vi "ActiView806-Lores.vi"() -> ()   [LabVIEW 2020] (continued)
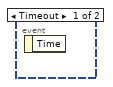
[diagram p2: hidden frame]
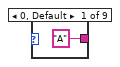
[diagram p3: hidden frame]
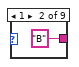
[diagram p4: hidden frame]
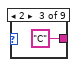
[diagram p5: hidden frame]
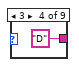
[diagram p6: hidden frame]
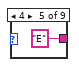
[diagram p7: hidden frame]
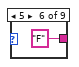
[diagram p8: hidden frame]
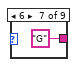
[diagram p9: hidden frame]
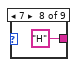
[diagram p10: hidden frame]
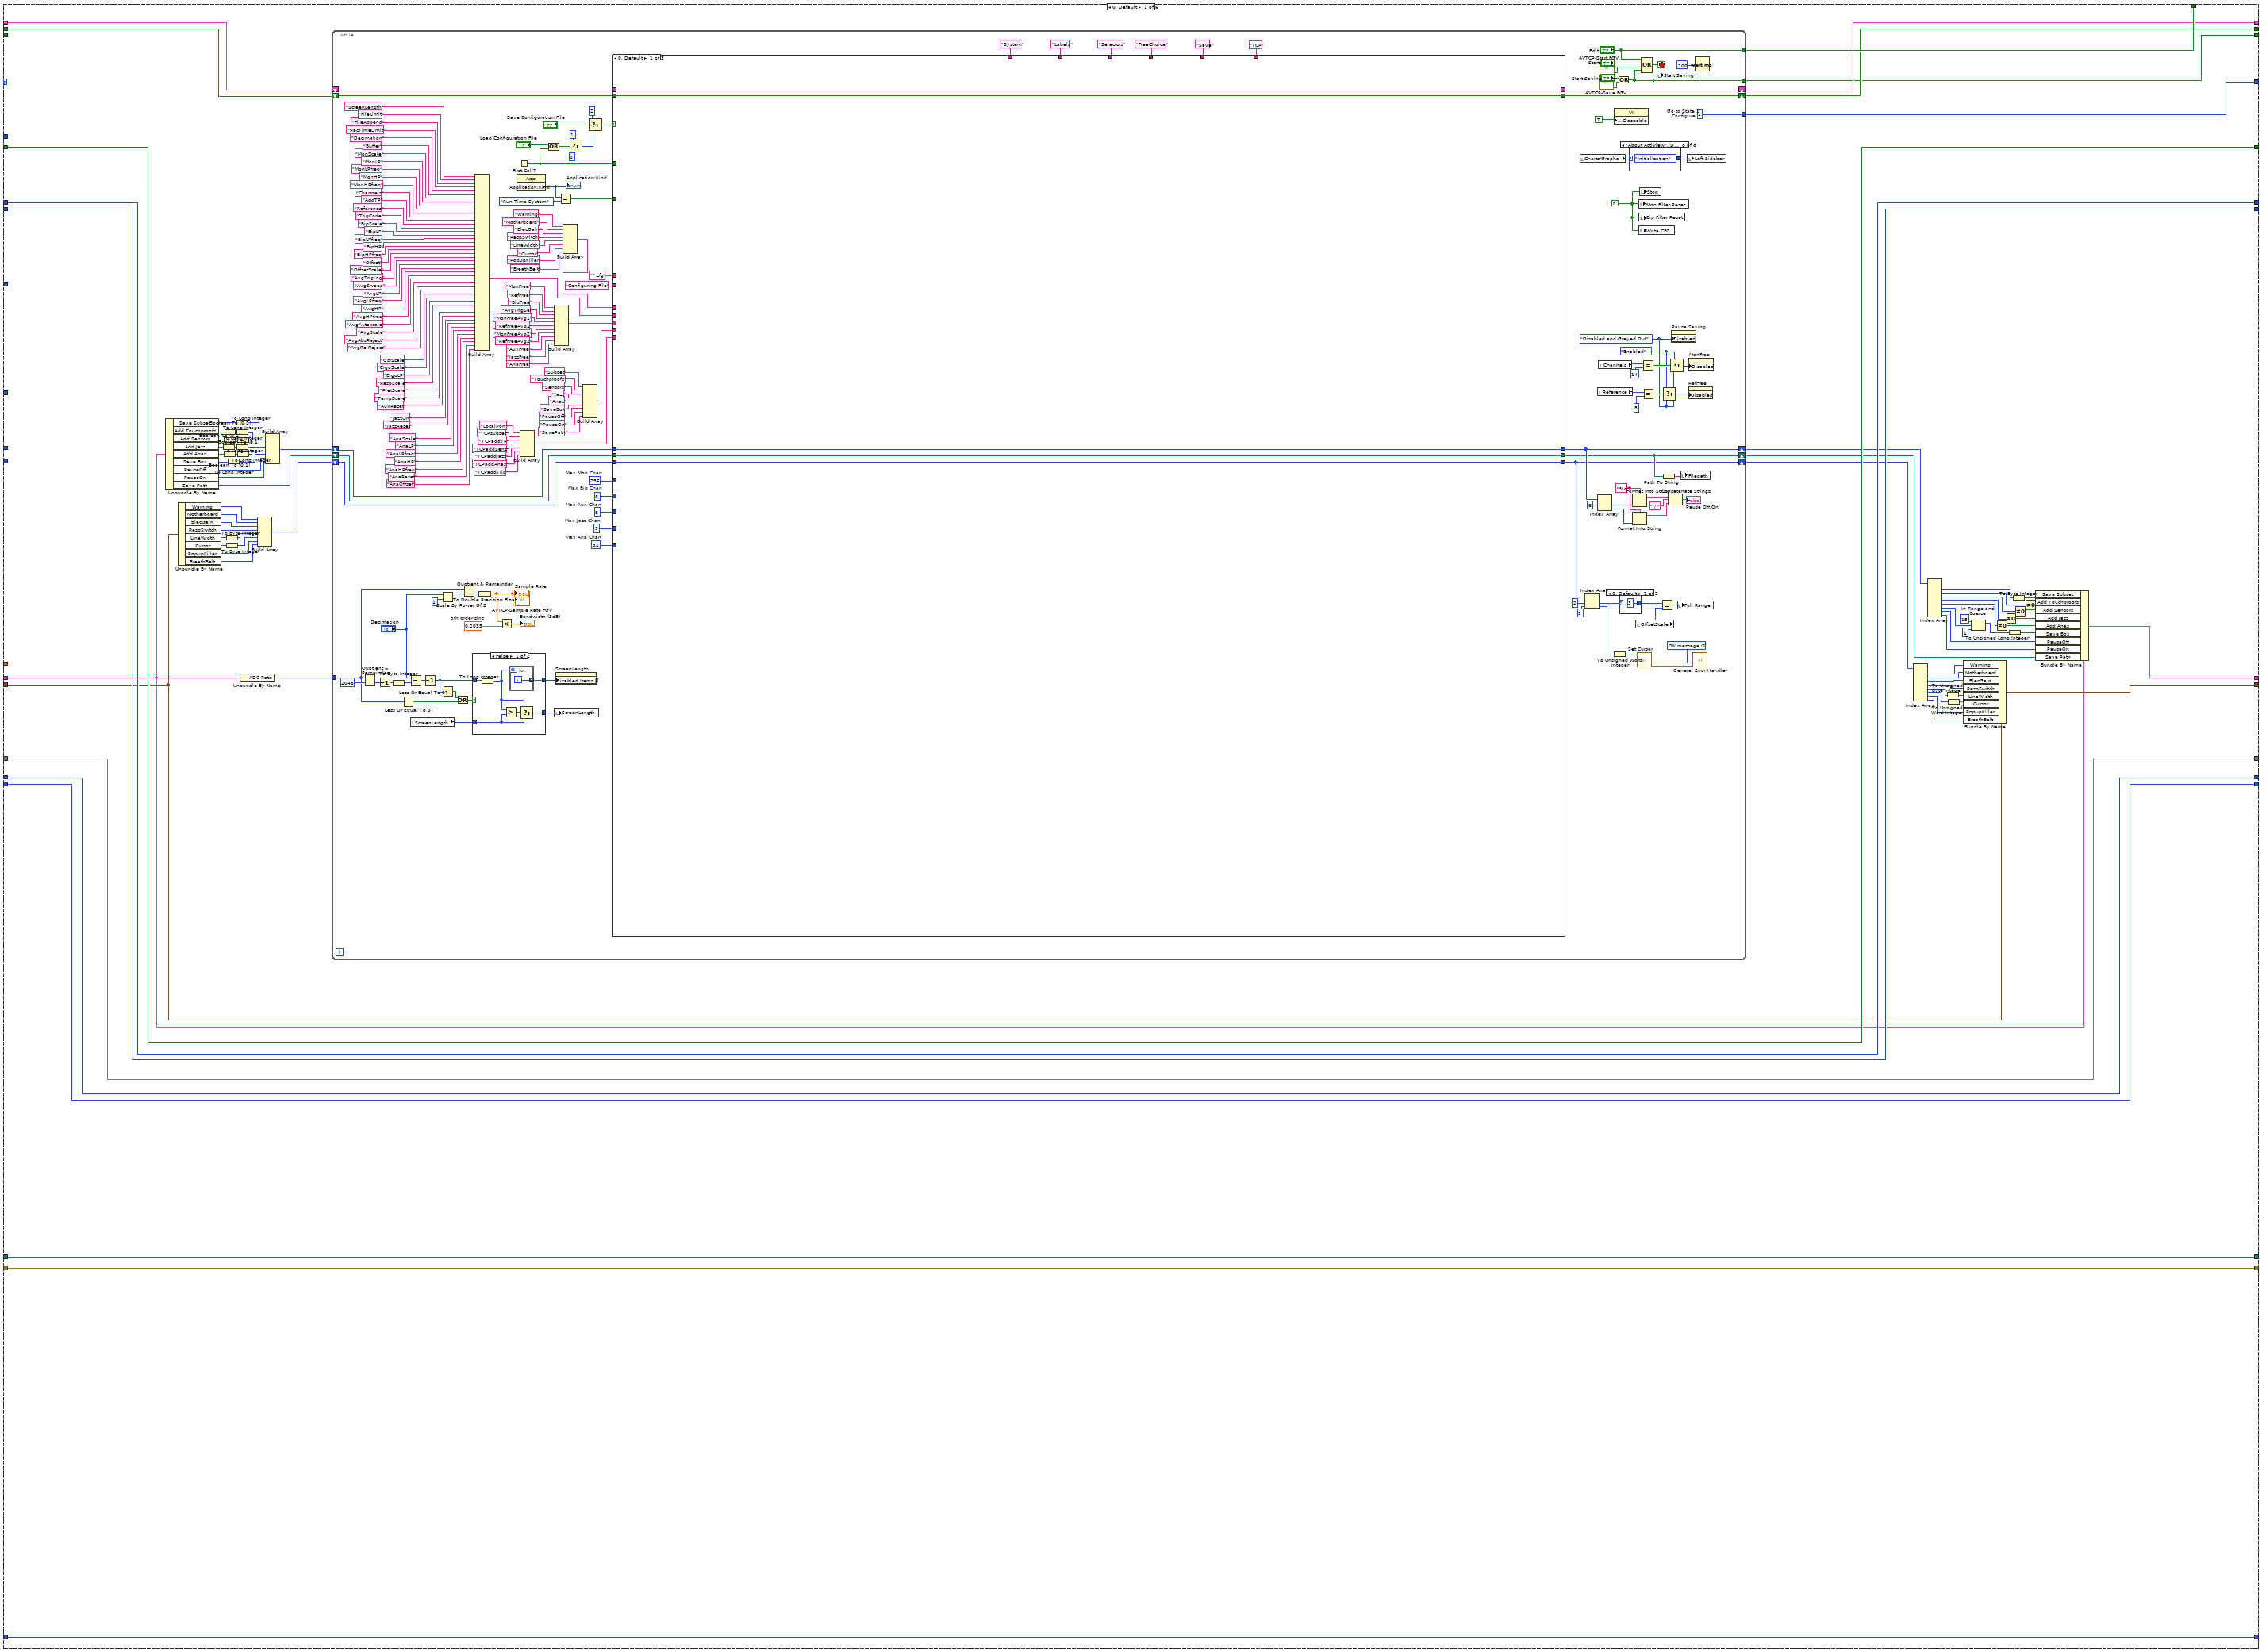
[diagram p11: hidden frame]
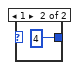
[diagram p12: hidden frame]
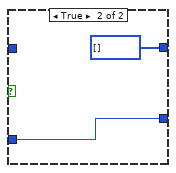
[diagram p13: hidden frame]
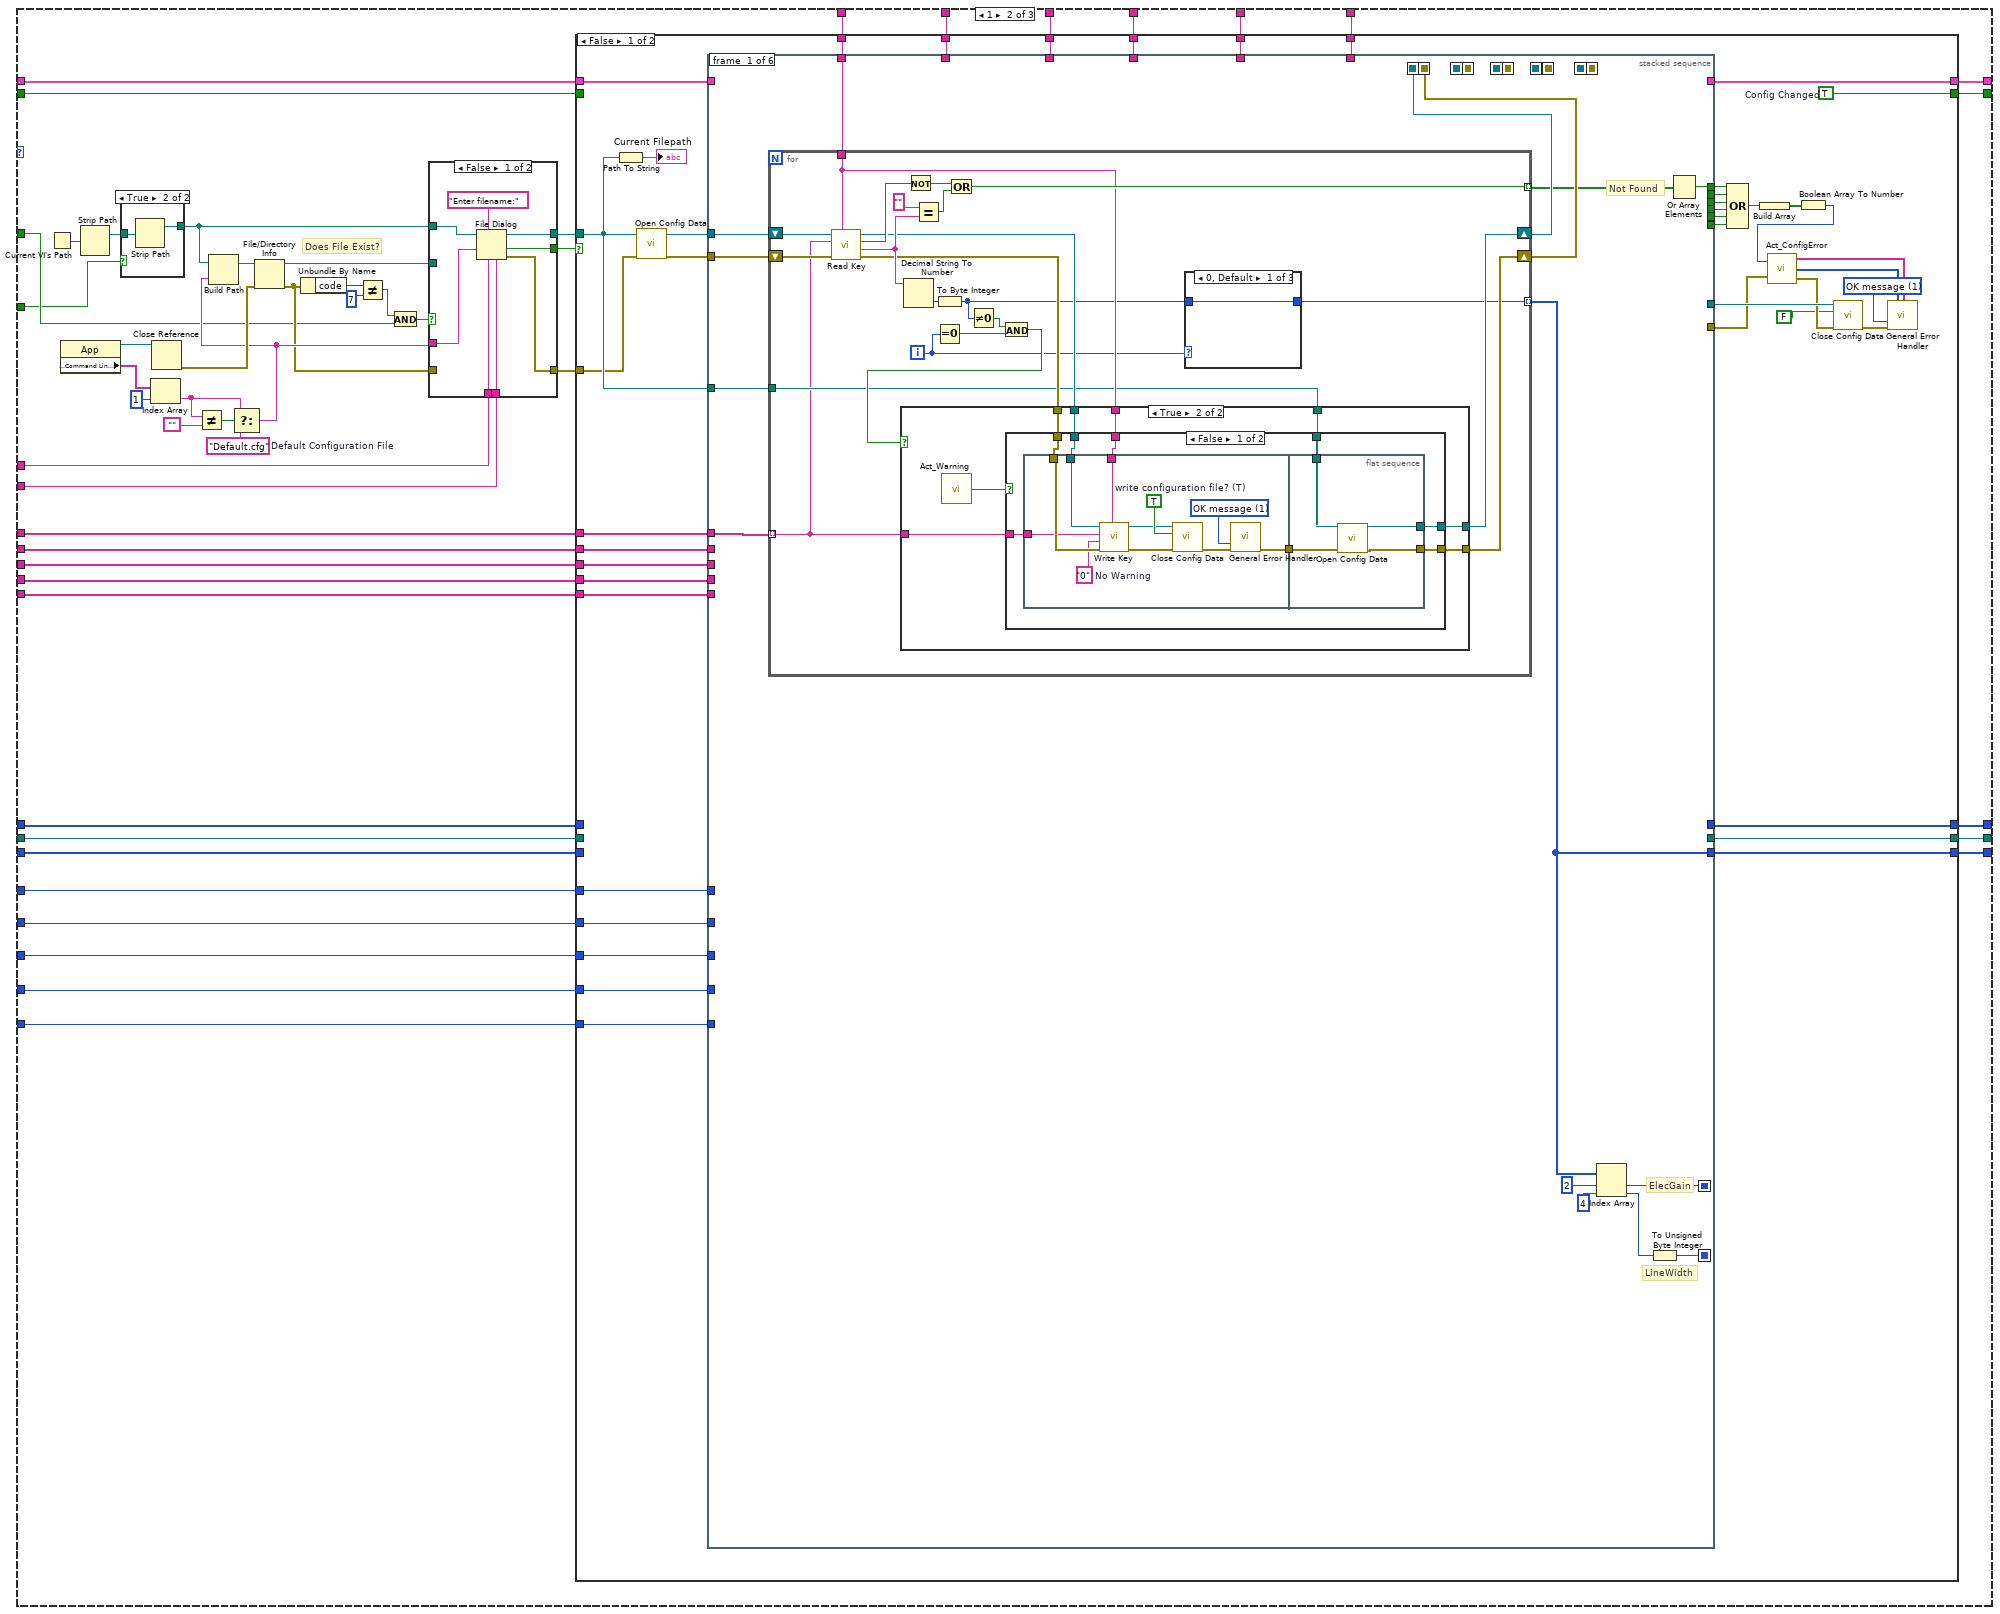
[diagram p14: hidden frame]
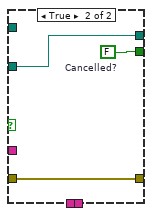
[diagram p15: hidden frame]
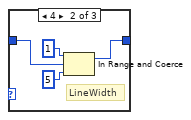
[diagram p16: hidden frame]
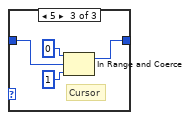
[diagram p17: hidden frame]
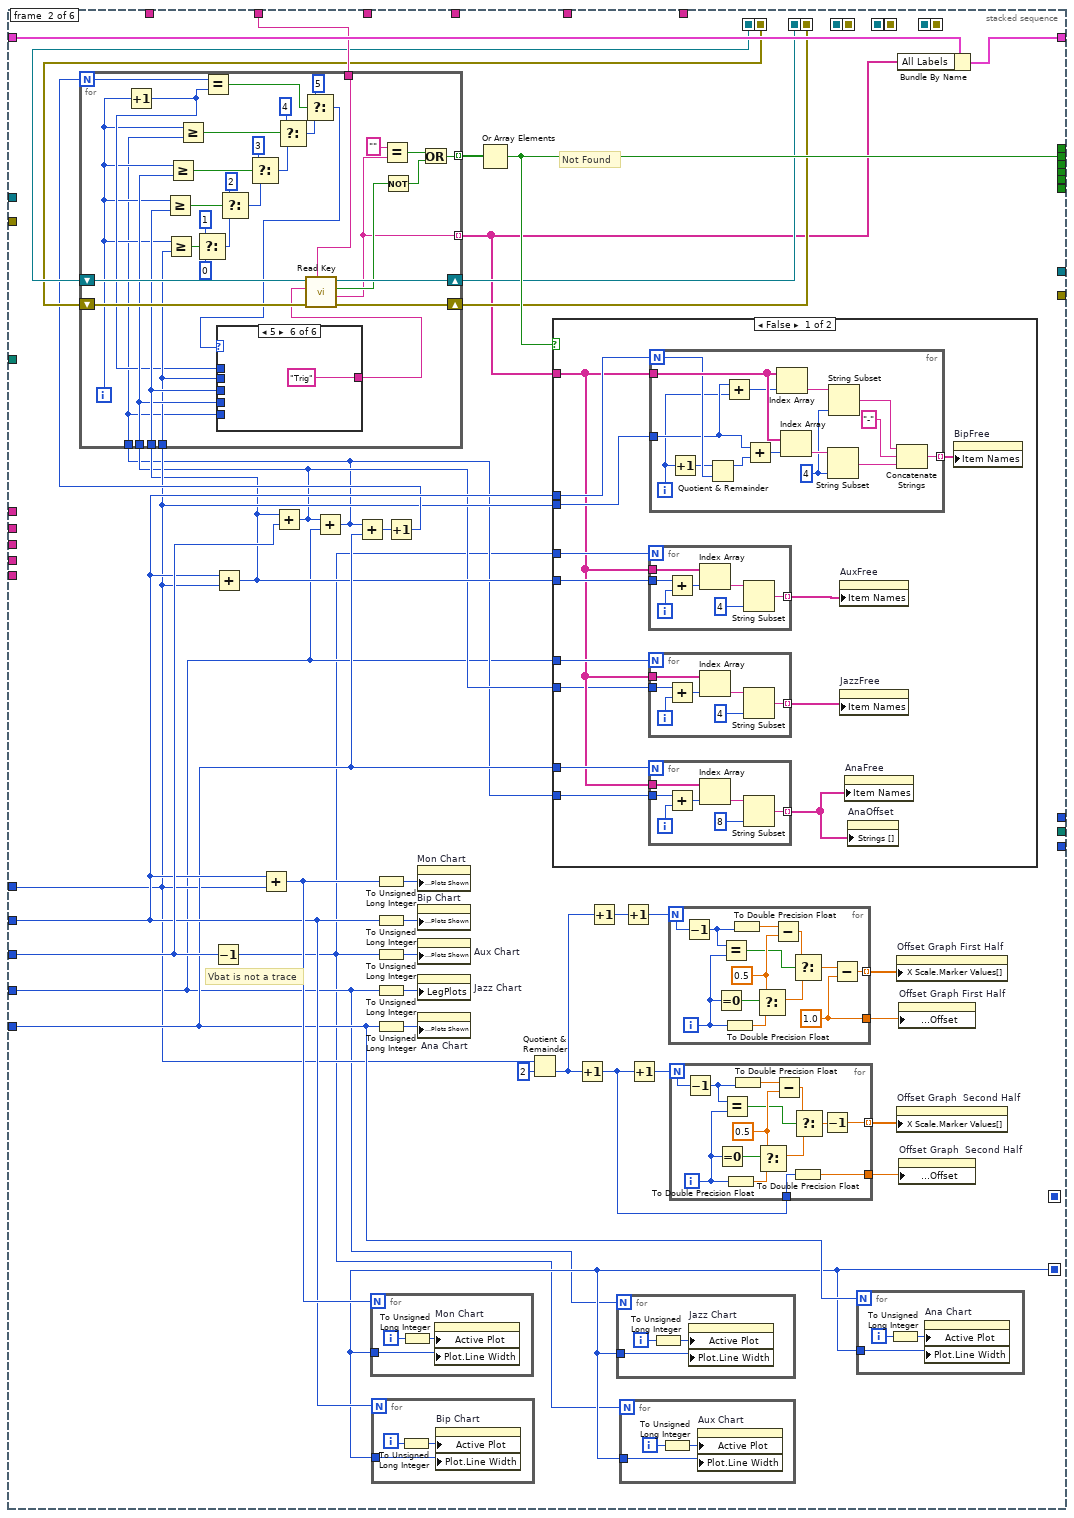
[diagram p20: hidden frame]
                          }
                        }
                      }
                    }
                    n2166 = property on="Avg2" class="WFGraph (strict)"("Y Scale.Range:Maximum"=w5030, "YScale.Minimum"=w5029) -> ()  [unwired: 2 in, 2 out]
                    "Avg2" <- w5031
                  }
                }
              }
            }
          }
          "Nr of Files" <- w2840
          n2167 = Unbundle By Name(w2940) -> ("Clear Block"=w2942:i32, "Screen Ratio"=w2941:dbl, "Y1"=w2938:i16, "Y2"=w2936:i16, "Y3"=w2937:i16, "Color"=w2939:u32)
          n2168 = case shown="True" w2951 {
            tunnel: w2964 -> [_ w3216]
            tunnel: w2907 -> [_ w3217]
            tunnel: w2965 -> [_ w3215]
            tunnel: w2802 -> [_ w3213]
            tunnel: w2966 -> [_ w3214]
            tunnel: w2967 -> [_ w3212]
            tunnel: w2959 -> [_ w3211]
            tunnel: w2944 -> [w3179 w3201]
            tunnel: [w3179 w3197] -> w2948
            tunnel: w2941 -> [_ w3208]
            tunnel: w2942 -> [_ w3207]
            tunnel: w2945 -> [w3178 w3204]
            tunnel: [w3178 w3195] -> w2947
            tunnel: w2943 -> [w3177 w3205]
            tunnel: [w3177 w3206] -> w2946
            tunnel: w2938 -> [_ w3199]
            tunnel: w2939 -> [_ w3193]
            tunnel: w2937 -> [_ w3191]
            tunnel: w2936 -> [_ w3189]
            tunnel: w2935 -> [_ w3182]
            tunnel: w2800 -> [_ w3187]
            frame False {
            }
            frame True {
              w3192 = TRUE ("fill?(F)")
              w3188 = i16 0
              n2169 = To Double Precision Float(number=w3216) -> (double precision float=w3180:dbl)
              n2170 = To Double Precision Float(number=w3217) -> (double precision float=w3181:dbl)
              n2171 = To Double Precision Float(number=w3207) -> (double precision float=w3210:dbl)
              n2172 = Divide(x=w3210, y=w3208) -> (x/y=w3209:dbl)
              n2173 = case shown="\"Monopolar Display\"" w3213 {
                tunnel: w3181 -> [w3231 w3238 w3248 w3260 w3271 _]
                tunnel: w3180 -> [w3232 w3239 w3250 w3261 w3272 _]
                tunnel: w3215 -> [w3230 _ _ _ _ _]
                tunnel: w3214 -> [_ w3237 _ _ _ _]
                tunnel: w3212 -> [_ _ w3249 _ _ _]
                tunnel: w3211 -> [_ _ _ _ w3270 _]
                tunnel: w3187 -> [_ _ _ w3259 _ _]
                frame "Monopolar Display" {
                  n2174 = Subtract(x=w3230, y=w3232) -> (x-y=w3226:dbl)
                  n2175 = Add(x=w3232, y=w3231) -> (x+y=w3228:dbl)
                  n2176 = Greater?(x=w3226, y=0.1) -> (0:w3227:bool)
                  n2177 = case shown="True" w3227 {
                    tunnel: w3232 -> [_ w3234]
                    tunnel: w3228 -> [_ w3233]
                    frame False {
                    }
                    frame True {
                      n2178 = stacked-sequence {
                        tunnel: w3234 -> [w3235 _]
                        tunnel: w3233 -> [_ w3236]
                        frame #0 {
                          n2179 = property on="Mon Chart" class="WFChart (strict)"("X Scale.Range:Minimum"=w3235) -> ()  [unwired: 2 in, 2 out]
                        }
                        frame #1 {
                          n2180 = property on="Mon Chart" class="WFChart (strict)"("X Scale.Range:Maximum"=w3236) -> ()  [unwired: 2 in, 2 out]
                        }
                      }
                    }
                  }
                }
                frame "Bipolar Leads" {
                  n2181 = Subtract(x=w3237, y=w3239) -> (x-y=w3240:dbl)
                  n2182 = Add(x=w3239, y=w3238) -> (x+y=w3242:dbl)
                  n2183 = Greater?(x=w3240, y=0.1) -> (0:w3241:bool)
                  n2184 = case shown="True" w3241 {
                    tunnel: w3239 -> [_ w3245]
                    tunnel: w3242 -> [_ w3244]
                    frame False {
                    }
                    frame True {
                      n2185 = stacked-sequence {
                        tunnel: w3245 -> [w3246 _]
                        tunnel: w3244 -> [_ w3247]
                        frame #0 {
                          n2186 = property on="Bip Chart" class="WFChart (strict)"("X Scale.Range:Minimum"=w3246) -> ()  [unwired: 2 in, 2 out]
                        }
                        frame #1 {
                          n2187 = property on="Bip Chart" class="WFChart (strict)"("X Scale.Range:Maximum"=w3247) -> ()  [unwired: 2 in, 2 out]
                        }
                      }
                    }
                  }
                }
                frame "Auxiliary Sensors" {
                  n2188 = Subtract(x=w3249, y=w3250) -> (x-y=w3251:dbl)
                  n2189 = Add(x=w3250, y=w3248) -> (x+y=w3253:dbl)
                  n2190 = Greater?(x=w3251, y=0.1) -> (0:w3252:bool)
                  n2191 = case shown="True" w3252 {
                    tunnel: w3250 -> [_ w3255]
                    tunnel: w3253 -> [_ w3256]
                    frame False {
                    }
                    frame True {
                      n2192 = stacked-sequence {
                        tunnel: w3255 -> [w3257 _]
                        tunnel: w3256 -> [_ w3258]
                        frame #0 {
                          n2193 = property on="Aux Chart" class="WFChart (strict)"("X Scale.Range:Minimum"=w3257) -> ()  [unwired: 2 in, 2 out]
                        }
                        frame #1 {
                          n2194 = property on="Aux Chart" class="WFChart (strict)"("X Scale.Range:Maximum"=w3258) -> ()  [unwired: 2 in, 2 out]
                        }
                      }
                    }
                  }
                }
                frame "Jazz Eyetracker" {
                  n2195 = Subtract(x=w3259, y=w3261) -> (x-y=w3262:dbl)
                  n2196 = Add(x=w3261, y=w3260) -> (x+y=w3264:dbl)
                  n2197 = Greater?(x=w3262, y=0.1) -> (0:w3263:bool)
                  n2198 = case shown="True" w3263 {
                    tunnel: w3261 -> [_ w3266]
                    tunnel: w3264 -> [_ w3267]
                    frame False {
                    }
                    frame True {
                      n2199 = stacked-sequence {
                        tunnel: w3266 -> [w3268 _]
                        tunnel: w3267 -> [_ w3269]
                        frame #0 {
                          n2200 = property on="Jazz Chart" class="WFChart (strict)"("XScale.Minimum"=w3268) -> ()  [unwired: 2 in, 2 out]
                        }
                        frame #1 {
                          n2201 = property on="Jazz Chart" class="WFChart (strict)"("XScale.Maximum"=w3269) -> ()  [unwired: 2 in, 2 out]
                        }
                      }
                    }
                  }
                }
                frame "Analog Input Box" {
                  n2202 = Subtract(x=w3270, y=w3272) -> (x-y=w3273:dbl)
                  n2203 = Add(x=w3272, y=w3271) -> (x+y=w3275:dbl)
                  n2204 = Greater?(x=w3273, y=0.1) -> (0:w3274:bool)
                  n2205 = case shown="True" w3274 {
                    tunnel: w3272 -> [_ w3277]
                    tunnel: w3275 -> [_ w3278]
                    frame False {
                    }
                    frame True {
                      n2206 = stacked-sequence {
                        tunnel: w3277 -> [w3279 _]
                        tunnel: w3278 -> [_ w3280]
                        frame #0 {
                          n2207 = property on="Ana Chart" class="WFChart (strict)"("X Scale.Range:Minimum"=w3279) -> ()  [unwired: 2 in, 2 out]
                        }
                        frame #1 {
                          n2208 = property on="Ana Chart" class="WFChart (strict)"("X Scale.Range:Maximum"=w3280) -> ()  [unwired: 2 in, 2 out]
                        }
                      }
                    }
                  }
                }
                frame "About ActiView", Default {
                }
              }
              n2209 = To Word Integer(number=w3209) -> (16bit integer=w3190:i16)
              n2210 = case shown="False" w3205 {
                tunnel: w3204 -> [_ w3225]
                tunnel: [w3222 w3225] -> w3203
                tunnel: [w3223 w3224] -> w3202
                tunnel: w3201 -> [w3223 _]
                frame False {
                  n2211 = call "Empty Picture"() -> ("empty picture"=w3222:picture)
                }
                frame True {
                  n2212 = call "Empty Picture"() -> ("empty picture"=w3224:picture)
                }
              }
              n2213 = Bundle(w3188, w3188, w3190, "Y1"=w3199) -> (w3200:cluster{i16, i16, i16, "Y1":i16})  [unwired: 1 out]
              n2214 = Bundle(w3188, "Y2"=w3189, w3190, "Y3"=w3191) -> (w3194:cluster{i16, "Y2":i16, i16, "Y3":i16})  [unwired: 1 out]
              n2215 = Subtract(x=w3182, y=w3180) -> (x-y=w3185:dbl)
              n2216 = Add(x=w3180, y=w3181) -> (x+y=w3183:dbl)
              n2217 = Greater?(x=w3185, y=0.1) -> (0:w3184:bool)
              n2218 = case shown="True" w3184 {
                tunnel: w3180 -> [_ w3219]
                tunnel: w3183 -> [_ w3218]
                frame False {
                }
                frame True {
                  n2219 = stacked-sequence {
                    tunnel: w3219 -> [w3220 _]
                    tunnel: w3218 -> [_ w3221]
                    frame #0 {
                      n2220 = property on="Trigger Chart" class="WFChart (strict)"("X Scale.Range:Minimum"=w3220) -> ()  [unwired: 2 in, 2 out]
                    }
                    frame #1 {
                      n2221 = property on="Trigger Chart" class="WFChart (strict)"("X Scale.Range:Maximum"=w3221) -> ()  [unwired: 2 in, 2 out]
                    }
                  }
                }
              }
              n2222 = call <vilib>:"Draw Rect.vi"("picture"=w3203, "rect"=w3200, "fill?(F)"=w3192, "color(black)"=w3193) -> ("new picture"=w3196:picture)  [unwired: 1 in, 4 out]
              n2223 = call <vilib>:"Draw Rect.vi"("picture"=w3202, "rect"=w3200, "fill?(F)"=w3192, "color(black)"=w3193) -> ("new picture"=w3198:picture)  [unwired: 1 in, 4 out]
              n2224 = call <vilib>:"Draw Rect.vi"("picture"=w3196, "rect"=w3194, "fill?(F)"=w3192, "color(black)"=w3193) -> ("new picture"=w3195:picture)  [unwired: 1 in, 4 out]
              n2225 = Not(x=w3205) -> (.not. x?=w3206:bool)
              n2226 = call <vilib>:"Draw Rect.vi"("picture"=w3198, "rect"=w3194, "fill?(F)"=w3192, "color(black)"=w3193) -> ("new picture"=w3197:picture)  [unwired: 1 in, 4 out]
            }
          }
          n2227 = Exclusive Or(1:w2769, 2:w2768) -> (0:w2763:bool[])
          n2228 = Or Array Elements(Boolean array=w2763) -> (logical OR=w2762:bool)
          n2229 = case shown="True" w2762 {
            tunnel: w2769 -> [_ w3017]
            tunnel: w2765 -> [w3015 w3022]
            tunnel: [w3015 w3021] -> w2770
            tunnel: w2761 -> [_ w3020]
            frame False {
              # "Driver Handle"
            }
            frame True {
              n2230 = Unbundle By Name(w3020) -> ("Jazz Channels"=w3019:i32)
              n2231 = Not Equal To 0?(x=w3019) -> (x != 0?=w3018:bool)
              n2232 = Build Array (concatenate)(w3017, w3018) -> (w3016:bool[])
              n2233 = call "Act_Write.vi"("Triggers"=w3016, "Handle In"=w3022) -> ("Handle Out"=w3021:i64)
            }
          }
          n2234 = call "AVTCP-Stop FGV.vi"() -> ("Value out"=w2758:bool)  [unwired: 7 in]
          n2235 = Multiply(x=w2900, y=i64 4) -> (x*y=w2901:i64)
          n2236 = Compound Arithmetic op=OR(w2815, w2961, "Stop", w2758) -> (w2926:bool)
          n2237 = To Double Precision Float(number=w2901) -> (double precision float=w2919:dbl)
          n2238 = To Double Precision Float(number=w2764) -> (double precision float=w2918:dbl)
          n2239 = Divide(x=w2919, y=w2908) -> (x/y=w2921:dbl)
          n2240 = Divide(x=w2918, y=w2908) -> (x/y=w2920:dbl)
          n2241 = Bundle(w2921, w2920) -> (→"Ring Buffer":cluster{dbl, dbl})  [unwired: 1 out]
          "Total Saved sec" <- w2842
        }
        n2242 = call-poly <vilib>:"Close Input Device.vi"("error in (no error)"=w2633, "device ID"=w2634) -> ()  [unwired: 9 out]
        n2243 = case shown="True" w2611 {
          tunnel: w2614 -> [w2724 w2727]
          tunnel: [w2724 w2726] -> w2613
          tunnel: w2612 -> [_ w2725]
          frame False {
          }
          frame True {
            n2244 = TCP Close Connection(connection ID=w2725, error in (no error)=w2727) -> (error out=w2726:errorcluster)  [unwired: 2 out]
          }
        }
        n2245 = call "Act_Close.vi"("Handle In"=w2544) -> ()
        n2246 = Or(x=w2564, y=w2563) -> (x .or. y?=w2562:bool)
        n2247 = Select(t=w2705, s=w2564, f=w2703) -> (s? t:f=w2704:i32)
      }
      frame 5 {
        w5043 = T5."Enabled" ("Disabled")
        w5061 = 0  # Initially Nothing Saved
        w5073 = 0  # Stay in State 0:    stop running
        w5046 = FALSE
        w5074 = FALSE  # Sop Running
        # "Save Blocksize in Byte"
        # "Current File in Byte"
        # "Header Lenght in Byte"
        # "Busy Saving"
        # "Busy Saving"
        n2248 = property on="Buffer" class="Ring (strict)"("Disabled"=w5043) -> ()  [unwired: 2 in, 2 out]
        n2249 = property on="Downsample Ratio" class="Ring (strict)"("Disabled"=w5043) -> ()  [unwired: 2 in, 2 out]
        n2250 = property on="Load Configuration File" class="Bool"("Disabled"=w5043) -> ()  [unwired: 2 in, 2 out]
        n2251 = property on="Save Configuration File" class="Bool"("Disabled"=w5043) -> ()  [unwired: 2 in, 2 out]
        n2252 = property on="Edit" class="Bool"("Disabled"=w5043) -> ()  [unwired: 2 in, 2 out]
        n2253 = property on="Channels" class="Ring (strict)"("Disabled"=w5043) -> ()  [unwired: 2 in, 2 out]
        n2254 = property on="AuxFree" class="LstBox (strict)"("Disabled"=w5043) -> ()  [unwired: 2 in, 2 out]
        n2255 = property on="JazzFree" class="LstBox (strict)"("Disabled"=w5043) -> ()  [unwired: 2 in, 2 out]
        n2256 = property on="AnaFree" class="LstBox (strict)"("Disabled"=w5043) -> ()  [unwired: 2 in, 2 out]
        n2257 = property on="RefFreeAvg2" class="LstBox (strict)"("Disabled"=w5043) -> ()  [unwired: 2 in, 2 out]
        n2258 = property on="MonFreeAvg2" class="LstBox (strict)"("Disabled"=w5043) -> ()  [unwired: 2 in, 2 out]
        n2259 = property on="ScreenLength" class="Ring (strict)"("Disabled"=w5043) -> ()  [unwired: 2 in, 2 out]
        n2260 = property on="RefFreeAvg1" class="LstBox (strict)"("Disabled"=w5043) -> ()  [unwired: 2 in, 2 out]
        n2261 = property on="MonFreeAvg1" class="LstBox (strict)"("Disabled"=w5043) -> ()  [unwired: 2 in, 2 out]
        n2262 = property on="AvgLP" class="Bool (strict)"("Disabled"=w5043) -> ()  [unwired: 2 in, 2 out]
        n2263 = property on="AvgLPfreq" class="DigNum (strict)"("Disabled"=w5043) -> ()  [unwired: 2 in, 2 out]
        n2264 = property on="AvgHP" class="Bool (strict)"("Disabled"=w5043) -> ()  [unwired: 2 in, 2 out]
        n2265 = property on="AvgHPfreq" class="DigNum (strict)"("Disabled"=w5043) -> ()  [unwired: 2 in, 2 out]
        n2266 = property on="TCPaddTrig" class="Bool (strict)"("Disabled"=w5043) -> ()  [unwired: 2 in, 2 out]
        n2267 = property on="LocalPort" class="DigNum (strict)"("Disabled"=w5043) -> ()  [unwired: 2 in, 2 out]
        n2268 = property on="TCPsubset" class="Ring (strict)"("Disabled"=w5043) -> ()  [unwired: 2 in, 2 out]
        n2269 = property on="TCPaddTP" class="Bool (strict)"("Disabled"=w5043) -> ()  [unwired: 2 in, 2 out]
        n2270 = property on="TCPaddSens" class="Bool (strict)"("Disabled"=w5043) -> ()  [unwired: 2 in, 2 out]
        n2271 = property on="TCPaddAnas" class="Bool (strict)"("Disabled"=w5043) -> ()  [unwired: 2 in, 2 out]
        n2272 = property on="TCPaddJazz" class="Bool (strict)"("Disabled"=w5043) -> ()  [unwired: 2 in, 2 out]
        n2273 = property on="AvgTrigSel" class="LstBox (strict)"("Disabled"=w5043) -> ()  [unwired: 2 in, 2 out]
        n2274 = property on="AvgTrigLog" class="Ring (strict)"("Disabled"=w5043) -> ()  [unwired: 2 in, 2 out]
        n2275 = property on="AvgSweep" class="DigNum (strict)"("Disabled"=w5043) -> ()  [unwired: 2 in, 2 out]
        n2276 = case shown="True" w5067 {
          tunnel: w5071 -> [w5105 w5130]
          tunnel: w5069 -> [w5106 w5112]
          tunnel: [w5106 w5113] -> w5058
          tunnel: [w5105 w5109] -> w5070
          tunnel: w5068 -> [_ w5117]
          tunnel: w5072 -> [_ w5129]
          tunnel: w5060 -> [_ w5120]
          tunnel: w5046 -> [_ w5110]
          frame False {
            n2277 = local write "Start Saving"(FALSE ("Start Saving")) -> ()
          }
          frame True {
            w5109 = refnum<file> refnum  # Dummy Refnum
            w5115 = errorcluster {"status"=FALSE, "code"=0, "source"=""}  # No error
            # "number of data records"
            n2278 = To Quad Integer(1:w5117) -> (0:w5107:i64)
            n2279 = To Quad Integer(1:w5120) -> (0:w5108:i64)
            n2280 = Unbundle By Name(w5112) -> ("code"=w5119:i32)
            n2281 = Subtract(x=w5129, y=w5107) -> (x-y=w5128:i64)
            n2282 = Quotient & Remainder(x=w5128, y=w5108) -> (floor(x/y)=w5121:i64)  [unwired: 1 out]
            n2283 = Less?(x=w5119, y=5000) -> (x < y?=w5111:bool)
            n2284 = Format Into String(format string="%-8d", w5121) -> (resulting string=w5126:string)  [unwired: 2 in, 1 out]
            n2285 = Select(t=w5112, s=w5111, f=w5115) -> (s? t:f=w5116:errorcluster)
            n2286 = call "Write File+ [String].vi"("String"=w5126, "error in (no error)"=w5116, "pos offset (bytes:0)"=i64 236, "pos mode (rel. to end:1)"=enum16{"start", "end", "current"}."start", "refnum"=w5130) -> ("error out"=w5125:errorcluster, "dup refnum"=w5124:refnum<file>)  [unwired: 2 out]
            n2287 = flat-sequence {
              tunnel: w5110 -> [w5132]
              frame #0 {
                n2288 = property on="Start Saving" class="Bool (strict)"("Boolean Text.Text"="Initializing") -> ()  [unwired: 2 in, 2 out]
              }
              frame #1 {
                n2289 = local write "Start Saving"(w5132) -> ()
              }
              frame #2 {
                n2290 = property on="Start Saving" class="Bool (strict)"("Boolean Text.Text"="Start File") -> ()  [unwired: 2 in, 2 out]
              }
            }
            n2291 = Close File(refnum=w5124, error in=w5125) -> (error out=w5114:errorcluster)  [unwired: 1 out]
            n2292 = Select(t=w5114, s=w5111, f=w5112) -> (s? t:f=w5113:errorcluster)
            n2293 = local write "Pause Saving"(w5110) -> ()
          }
        }
        n2294 = flat-sequence {
          tunnel: w5045 -> [w5083]
          frame #0 {
            n2295 = Unbundle By Name(w5083) -> ("JazzRec"=w5080:bool, "Speed Mode"=w5078:i8)
            n2296 = Less Than 0?(x=w5078) -> (x < 0?=w5076:bool)
            n2297 = Greater?(x=w5078, y=i8 3) -> (0:w5081:bool)
            n2298 = Or(x=w5081, y=w5076) -> (x .or. y?=w5077:bool)
            n2299 = property on="Charts/Graphs" class="TabCtl (strict)"() -> ("Pages"=w5086:refnum<vi>[])  [unwired: 2 in, 2 out]
            n2300 = And(x=w5080, y=w5077) -> (x .and. y?=w5079:bool)
            n2301 = Index Array(array=w5086, index=5) -> (element=w5084:refnum<vi>)
            n2302 = Select(t=T4."Page Enabled" ("Page Enabled State"), s=w5079, f=T4."Page Disabled & Grayed" ("Page Enabled State")) -> (s? t:f=w5089:T4)
            n2303 = property class="Page"(reference=w5084, "Page Enabled State"=w5089) -> ()  [unwired: 1 in, 2 out]
          }
          frame #1 {
            n2304 = property on="JazzOn" class="Bool (strict)"("Disabled"=T5."Enabled") -> ()  [unwired: 2 in, 2 out]
          }
        }
        n2305 = local write "Write"(w5046) -> ()
        n2306 = local write "Start"(w5046) -> ()
        n2307 = local write "Averaging"(w5046) -> ()
        n2308 = local write "Sweeping"(w5046) -> ()
        n2309 = local write "TCP Connected"(w5046) -> ()
        n2310 = local write "TCP Listening"(w5046) -> ()
        n2311 = Unbundle By Name(w5058) -> ("code"=w5059:i32)
        n2312 = property on="Start Saving" class="Bool (strict)"() -> ("Colors [4]"=w5051:cluster{u32, u32}[])  [unwired: 2 in, 2 out]
        n2313 = case shown="0, Default" w5059 {
          tunnel: w5058 -> [w5092 w5101]
          tunnel: [w5099 w5100] -> w5057
          frame 0, Default {
            w5091 = T18 1 items=["no dialog", "OK message", "continue or stop message", "OK message + warnings", "continue/stop + warnings"] ("type of dialog (OK msg:1)")
            w5099 = errorcluster {"status"=FALSE, "code"=0, "source"=""}  # No Error
            n2314 = call "Act_Error_Jazz.vi"() -> ("[user-defined descriptions]"=w5093:string[], "[user-defined codes]"=w5096:i32[])  [unwired: 2 in, 1 out]
            n2315 = call "Act_ConfigError.vi"() -> ("[user-defined descriptions]"=w5094:string[], "[user-defined codes]"=w5098:i32[])  [unwired: 2 in, 1 out]
            n2316 = Build Array (concatenate)(w5093, w5094) -> (w5095:string[])
            n2317 = Build Array (concatenate)(w5096, w5098) -> (w5097:i32[])
            n2318 = call <vilib>:"General Error Handler.vi"("[user-defined codes]"=w5097, "[user-defined descriptions]"=w5095, "type of dialog (OK msg:1)"=w5091, "error in (no error)"=w5092) -> ()  [unwired: 1 in, 11 out]
          }
          frame 5003 {
            n2319 = call "Error to Warning.vi"("1st Error to Convert"=5003, "error in"=w5101) -> ("warning out"=w5103:errorcluster)  [unwired: 3 in, 10 out]
            n2320 = call "Display Message to User"("error in (no error)"=w5103) -> ("error out"=w5100:errorcluster)  [unwired: 2 in, 8 out]
          }
        }
        n2321 = Index Array(array=w5051) -> (element #1=w5053:cluster{u32, u32}, element #2=w5052:cluster{u32, u32})  [unwired: 2 in]
        n2322 = Unbundle(w5052) -> (w5054:u32)  [unwired: 1 out]
        n2323 = Bundle(u32 16724991, w5054) -> (w5055:cluster{u32, u32})  [unwired: 1 out]
        n2324 = Build Array(w5053, w5055) -> (w5049:cluster{u32, u32}[])
        n2325 = property on="Start Saving" class="Bool (strict)"("Colors [4]"=w5049, "Boolean Text.Text Colors:Text Color"=u32 16777215) -> ()  [unwired: 2 in, 2 out]
        n2326 = To Quad Integer(1:w5061) -> (0:w5044:i64)
      }
    }
  }
  n2327 = while {
    stop <- w5134 stop-if-true
    n2328 = event shown="[1] Panel Close?" {
      selector: _ -> [_ _]
      dyn-events: _ -> [_ _]
      timeout: _ -> [_ _]
      tunnel: [_ TRUE] -> w5134
      event Timeout {
        n2329 = event-data() -> ()  [unwired: 1 in, 1 out]
      }
      event Panel Close? {
        n2330 = event-data() -> ()  [unwired: 1 in, 1 out]
        n2331 = call "Logger-Close Log.vi"() -> ()  [unwired: 15 in, 1 out]
        n2332 = event-data("Discard?"=FALSE) -> ()  [unwired: 1 in, 1 out]
      }
    }
  }
